vi "Handle RESULT.vi"(0 "reference":refnum<class "WAMP Client.lvclass">, 5 "error in (no error)":errorcluster, 7 "WAMP Message":T3 {"Message Codes" items=["HELLO"=1, "WELCOME"=2, "ABORT"=3, "GOODBYE"=6, "ERROR"=8, "PUBLISH"=16, "PUBLISHED"=17, "SUBSCRIBE"=32, "SUBSCRIBED"=33, "UNSUBSCRIBE"=34, "UNSUBSCRIBED"=35, "EVENT"=36, "CALL"=48, "RESULT"=59, "REGISTER"=64, "REGISTERED"=65, "UNREGISTER"=66, "UNREGISTERED"=67, "INVOCATION"=68, "YIELD"=70]}, 9 "Call Requests":T1) -> (4 "reference out":refnum<class "WAMP Client.lvclass">, 6 "error out":errorcluster, 10 "map out":T1)   [LabVIEW 2020, in "WAMP Client.lvclass"]
uses:
  <userlib>/lvwamp/WAMP Client/WAMP Client.lvclass
  <userlib>/lvwamp/WAMP Client/TypeDef/WAMP Received Message.ctl
  <userlib>/lvwamp/WAMP Message Codes.ctl
  <userlib>/lvwamp/WAMP Client/TypeDef/CALL Request Map.ctl
  <userlib>/lvwamp/WAMP Client/TypeDef/CALL Request Data.ctl
  <userlib>/lvwamp/WAMP Client/TypeDef/RESULT Payload.ctl
  <userlib>/lvwamp/WAMP Client/TypeDef/WAMP Error Payload.ctl
  <userlib>/lvwamp/WAMP Client/WAMP Client.lvclass/WAMP Client.ctl
  <vilib>/JDP Science/JSONtext/JSONtext.lvlib
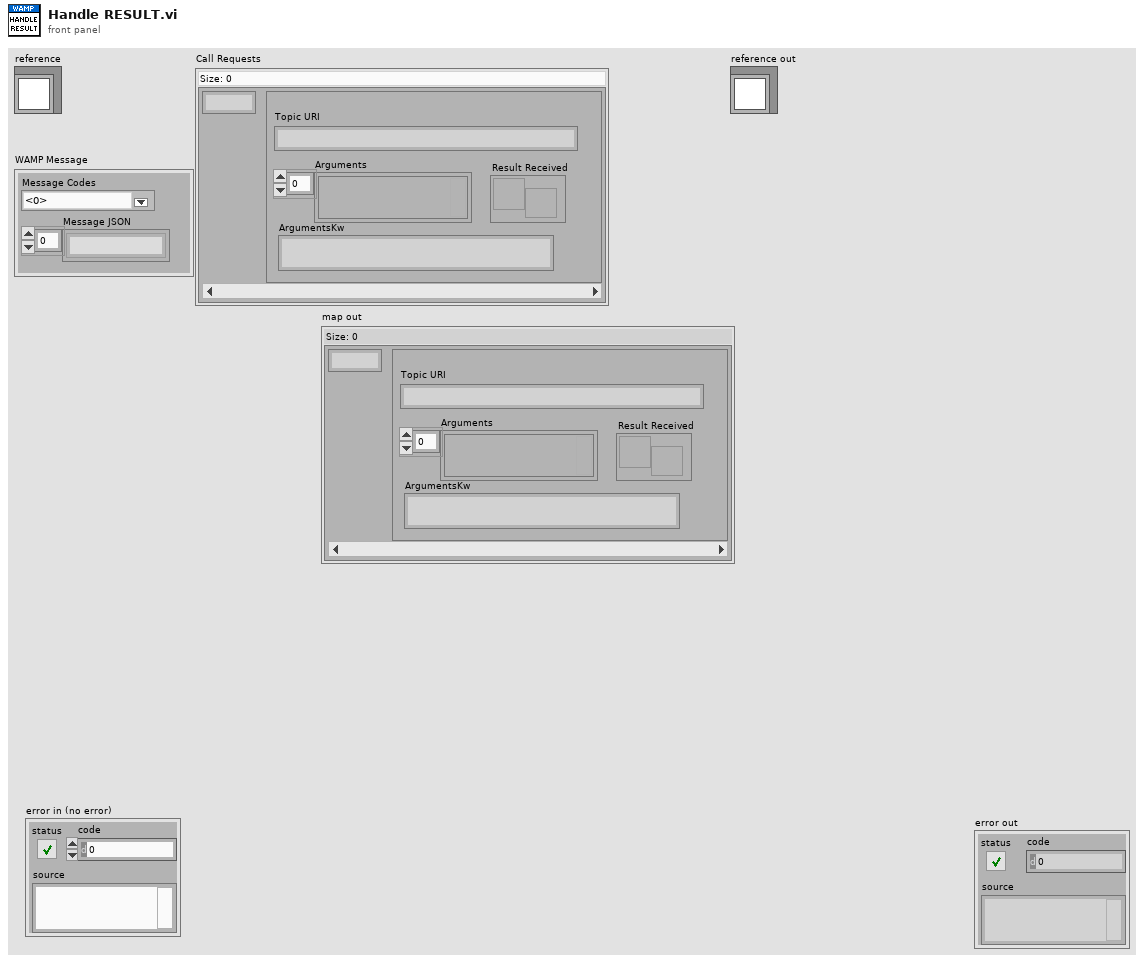
[diagram p1: front panel]
types:
  T1 = typedef "WAMP Client.lvclass/CALL Request Map.ctl" = map{u32, T2}
  T2 = typedef "WAMP Client.lvclass/CALL Request Data.ctl" = cluster{"Topic URI":string, "Arguments":variant[], "ArgumentsKw":string, "Result Received":refnum<user-event>}
  T3 = typedef "WAMP Client.lvclass/WAMP Received Message.ctl" = cluster{"Message JSON":string[], "Message Codes":T4}
  T4 = typedef "WAMP Client.lvclass/WAMP Message Codes.ctl" = u16
  T5 = typedef "WAMP Client.lvclass/RESULT Payload.ctl" = cluster{"Arguments Payload":string[], "ArgumentKw Payload":string, "Topic":string, "Success?":bool, "WAMP Error":T6}
  T6 = typedef "WAMP Client.lvclass/WAMP Error Payload.ctl" = cluster{"Arguments Payload":string[], "ArgumentKw Payload":string, "Error URI":string, "Error?":bool}
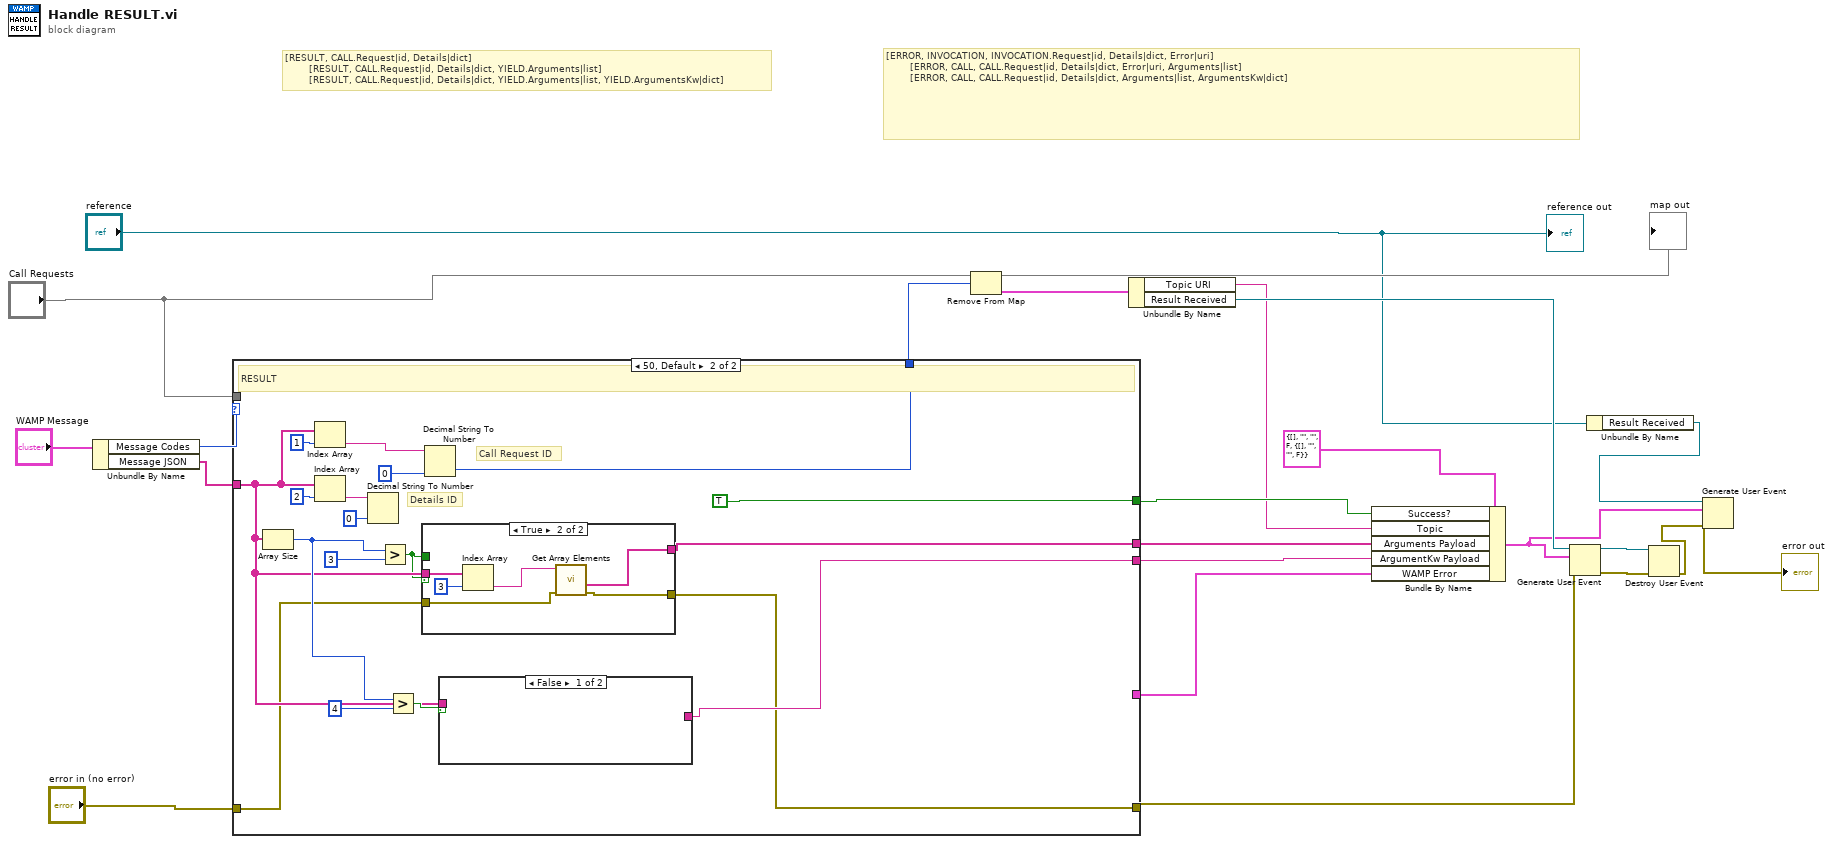
[diagram p0: block diagram]
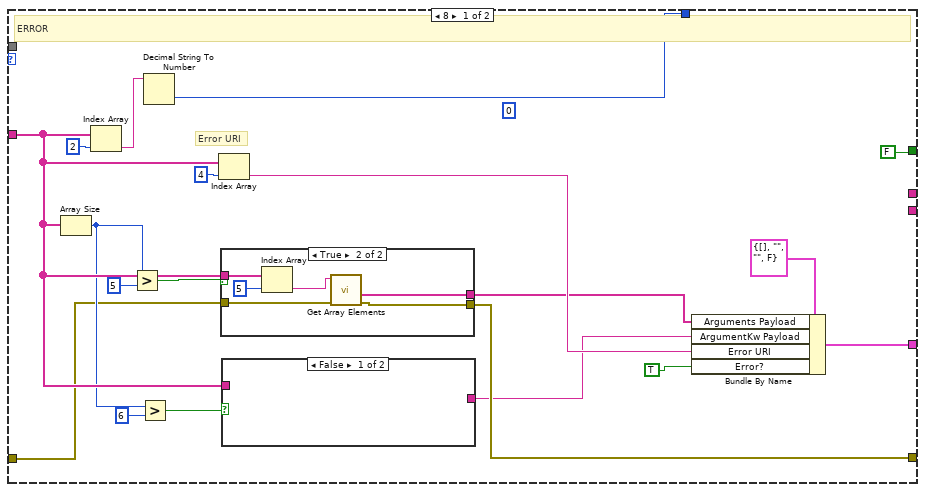
[diagram p2: hidden frame]
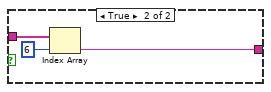
[diagram p3: hidden frame]
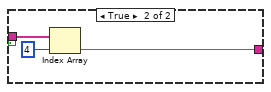
[diagram p5: hidden frame]
diagram:
  # "[ERROR, INVOCATION, INVOCATION.Request|id, Details|dict, Error|uri]\n        [ERROR, CALL, CALL.Request|id, Details|dict, Error|uri, Arguments|list]\n        [ERROR, CALL, CALL.Request|id, Details|dict, Arguments|list, ArgumentsKw|dict]"
  # "[RESULT, CALL.Request|id, Details|dict]\n        [RESULT, CALL.Request|id, Details|dict, YIELD.Arguments|list]\n        [RESULT, CALL.Request|id, Details|dict, YIELD.Arguments|list, YIELD.ArgumentsKw|dict]"
  n1 = Unbundle By Name("WAMP Message") -> ("Message Codes"=w19:T4, "Message JSON"=w18:string[])
  n2 = case shown="50, Default" w19 {
    tunnel: w18 -> [w35 w57]
    tunnel: [w38 w54] -> w17
    tunnel: "error in (no error)" -> [w31 w56]
    tunnel: [w30 w55] -> w21
    tunnel: [FALSE ("Success?") TRUE ("Success?")] -> w22
    tunnel: "Call Requests" -> [_ _]
    tunnel: [_ w59] -> w11
    tunnel: [_ w58] -> w10
    tunnel: [w24 _] -> w1
    frame 8 {
      (unwired) 0
      # "Error URI"
      # "ERROR"
      n3 = Array Size(array=w35) -> (size(s)=w32:i32)
      n4 = Index Array(array=w35, index=2) -> (element=w41:string)
      n5 = Greater?(x=w32, y=5) -> (0:w36:bool)
      n6 = Greater?(x=w32, y=6) -> (0:w33:bool)
      n7 = Decimal String To Number(string=w41) -> (number=w38:i32)  [unwired: 2 in, 1 out]
      n8 = Index Array(array=w35, index=4) -> (element=w27:string)
      n9 = case shown="True" w36 {
        tunnel: w35 -> [_ w51]
        tunnel: [_ w50] -> w26
        tunnel: w31 -> [w46 w48]
        tunnel: [w46 w47] -> w30
        frame False {
        }
        frame True {
          n10 = Index Array(array=w51, index=5) -> (element=w49:string)
          n11 = call <vilib>:"Get Array Elements.vi"("error in (no error)"=w48, "JSON"=w49) -> ("error out"=w47:errorcluster, "<JSON>"=w50:string[])  [unwired: 7 in, 1 out]
        }
      }
      n12 = case shown="False" w33 {
        tunnel: [_ w44] -> w25
        tunnel: w35 -> [_ w43]
        frame False {
        }
        frame True {
          n13 = Index Array(array=w43, index=6) -> (element=w44:string)
        }
      }
      n14 = Bundle By Name(cluster=T6 {"Arguments Payload"=[], "ArgumentKw Payload"="", "Error URI"="", "Error?"=FALSE} ("Cluster"), "Arguments Payload"=w26, "ArgumentKw Payload"=w25, "Error URI"=w27, "Error?"=TRUE ("status")) -> (w24:T6)
    }
    frame 50, Default {
      # "Call Request ID"
      # "Details ID"
      # "RESULT"
      n15 = Array Size(array=w57) -> (size(s)=w60:i32)
      n16 = Index Array(array=w57, index=1) -> (element=w66:string)
      n17 = Index Array(array=w57, index=2) -> (element=w69:string)
      n18 = Decimal String To Number(string=w69, default (0L)=u32 0) -> ()  [unwired: 1 in, 2 out]
      n19 = Greater?(x=w60, y=3) -> (0:w53:bool)
      n20 = Greater?(x=w60, y=4) -> (0:w61:bool)
      n21 = case shown="True" w53 {
        tunnel: w53 -> [_ _]
        tunnel: [_ w79] -> w59
        tunnel: [w74 w78] -> w55
        tunnel: w57 -> [_ w77]
        tunnel: w56 -> [w74 w75]
        frame False {
        }
        frame True {
          n22 = Index Array(array=w77, index=3) -> (element=w76:string)
          n23 = call <vilib>:"Get Array Elements.vi"("error in (no error)"=w75, "JSON"=w76) -> ("error out"=w78:errorcluster, "<JSON>"=w79:string[])  [unwired: 7 in, 1 out]
        }
      }
      n24 = Decimal String To Number(string=w66, default (0L)=u32 0) -> (number=w54:u32)  [unwired: 1 in, 1 out]
      n25 = case shown="False" w61 {
        tunnel: [_ w72] -> w58
        tunnel: w57 -> [_ w71]
        frame False {
        }
        frame True {
          n26 = Index Array(array=w71, index=4) -> (element=w72:string)
        }
      }
    }
  }
  n27 = Remove From Map(10:w17, 11:"Call Requests") -> (1:w16:T2, 3:→"map out":T1)  [unwired: 1 out]
  n28 = Unbundle By Name(w16) -> ("Topic URI"=w8:string, "Result Received"=w9:refnum<user-event>)
  n29 = Bundle By Name(cluster=T5 {"Arguments Payload"=[], "ArgumentKw Payload"="", "Topic"="", "Success?"=FALSE, "WAMP Error"={"Arguments Payload"=[], "ArgumentKw Payload"="", "Error URI"="", "Error?"=FALSE}} ("RESULT Payload"), "Success?"=w22, "Topic"=w8, "Arguments Payload"=w11, "ArgumentKw Payload"=w10, "WAMP Error"=w1) -> (w5:T5)
  n30 = Generate User Event(user event=w9, event data cluster=w5, error in=w21) -> (user event out=w14:refnum<user-event>, error out=w15:errorcluster)  [unwired: 1 in]
  n31 = Unbundle By Name("reference") -> ("Result Received"=w4:refnum<user-event>)
  n32 = Destroy User Event(user event=w14, error in=w15) -> (error out=w3:errorcluster)
  n33 = Generate User Event(user event=w4, event data cluster=w5, error in=w3) -> (error out=→"error out":errorcluster)  [unwired: 1 in, 1 out]
  "reference out" <- "reference"
